vi "ESP301.vi"() -> ()   [LabVIEW 2019]
uses:
  Newport ESP301/Newport ESP301.lvlib
panel:
  in  "DigNum Refnum":refnum<vi>
  out "Numeric":i32
  out "Left Travel Limit (units)":dbl format="%.6g"
  out "Right Travel Limit (units)":dbl format="%.6g"
  in  "Power Status":bool
  out "Units":T1(ring)
  in  "Target position (units)":dbl
  in  "Stop":bool
  out "Position (units)":dbl format="%.6g"
  out "Home High Speed (units/s)":dbl format="%.4g"
  out "Maximum Velocity (units/s)":dbl format="%.4g"
  out "Velocity (units/s)":dbl format="%.4g"
  in  "VISA resource name":refnum<visa-resource-name>
  in  "Axis (1)":i32=1 min=1 max=3
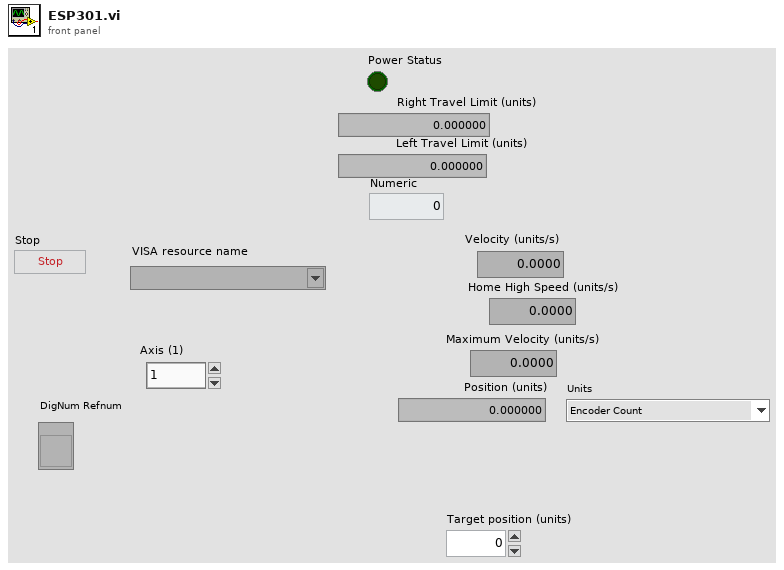
[diagram p1: front panel]
types:
  T1 = enum16{"Encoder Count", "Motor Step", "millimeter", "micrometer", "inch", "milli-inch", "micro-inch", "degree", "gradian", "radian", "milliradian", "microradian"}
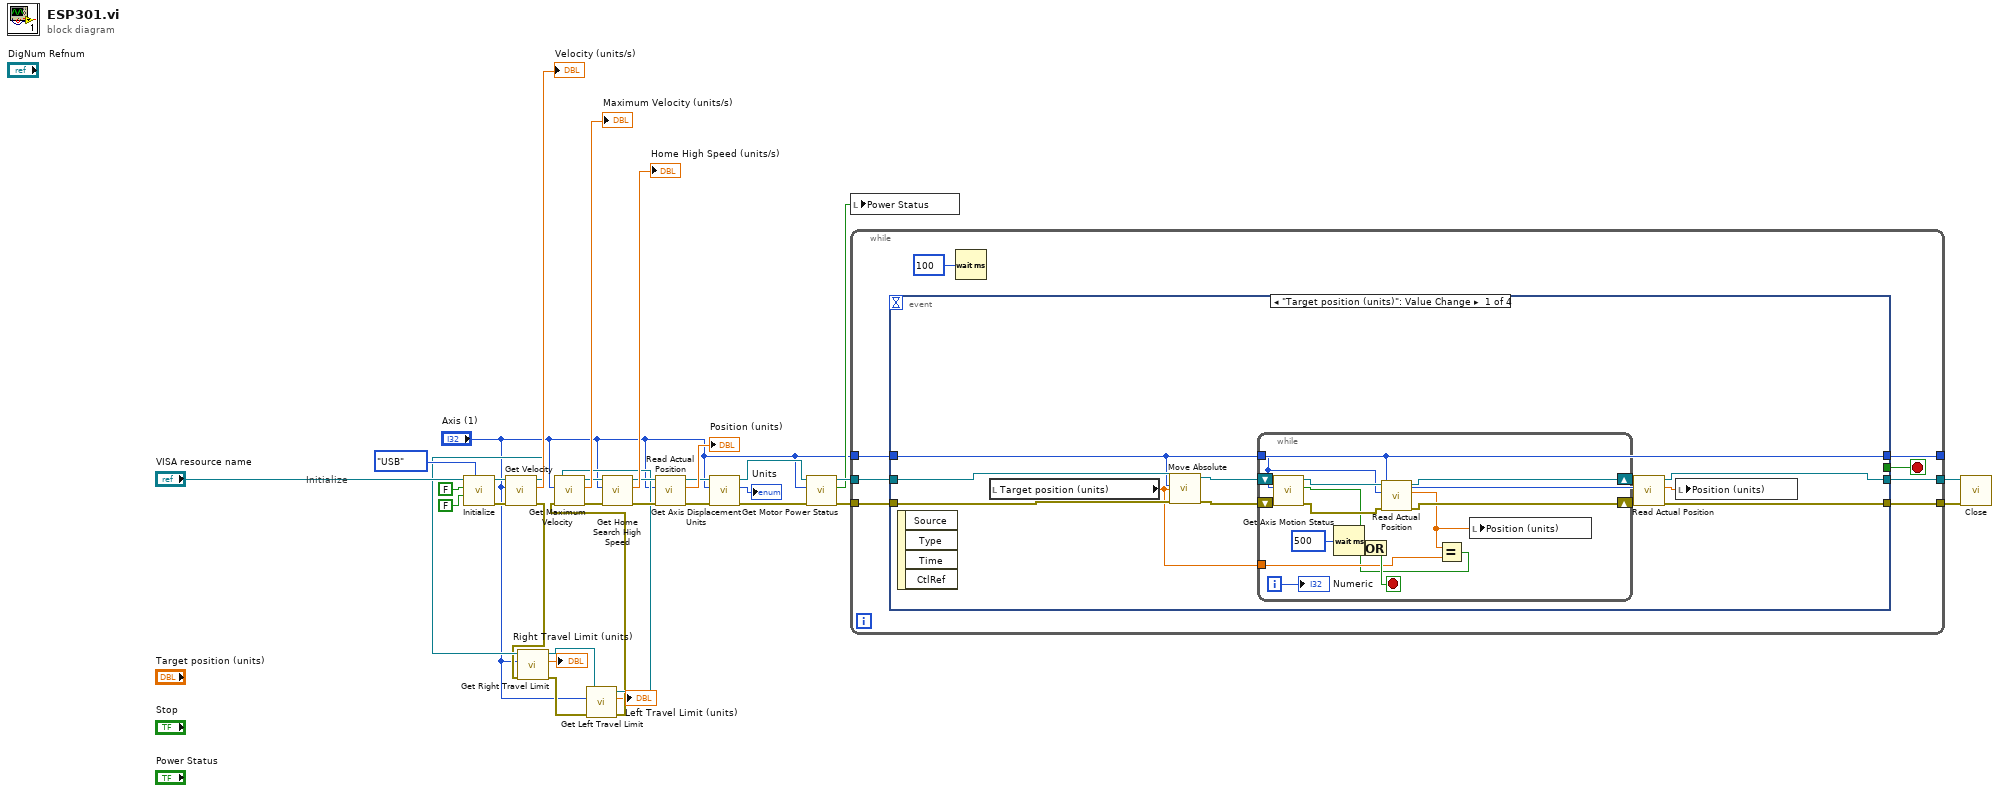
[diagram p0: block diagram]
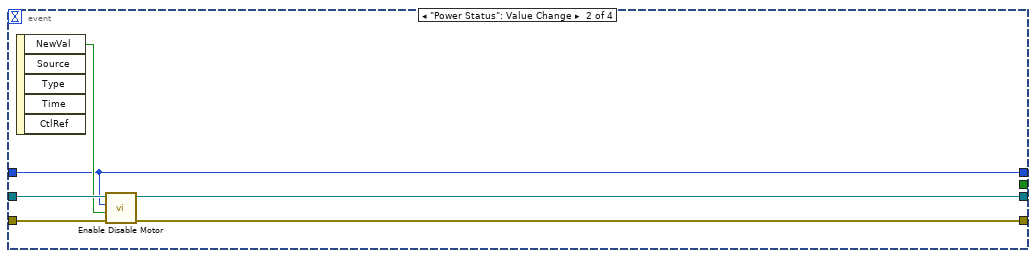
[diagram p2: hidden frame]
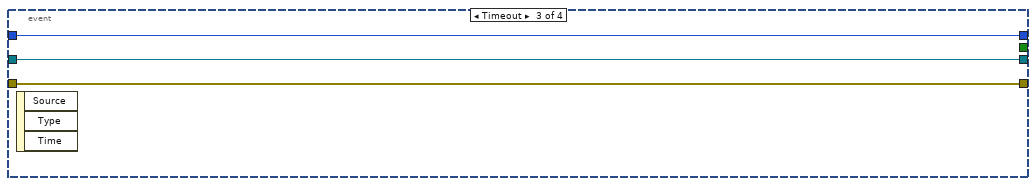
[diagram p3: hidden frame]
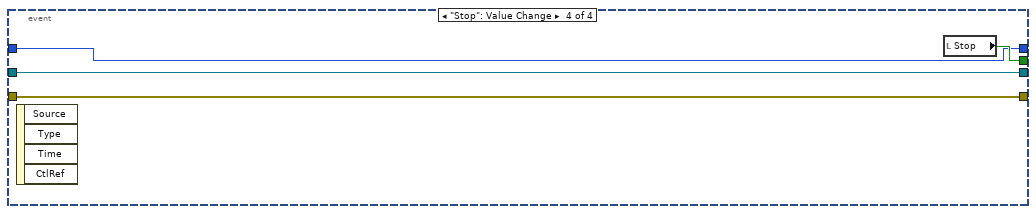
[diagram p4: hidden frame]
diagram:
  # "Initialize"
  n1 = call "Initialize.vi"("VISA resource name"="VISA resource name", "ID Query (True)"=FALSE, "Reset (False)"=FALSE, "Serial Link (RS232)"=enum16{"RS232", "USB"}."USB") -> ("VISA resource name out"=w32:refnum<visa-resource-name>, "error out"=w31:errorcluster)  [unwired: 5 in]
  n2 = call "Get Velocity.vi"("error in (no error)"=w31, "Axis (1)"="Axis (1)", "VISA resource name"=w32) -> ("error out"=w8:errorcluster, "Velocity (units/s)"=→"Velocity (units/s)":dbl, "VISA resource name out"=w9:refnum<visa-resource-name>)  [unwired: 2 in]
  n3 = call "Get Right Travel Limit.vi"("error in (no error)"=w8, "Axis (1)"="Axis (1)", "VISA resource name"=w9) -> ("error out"=w5:errorcluster, "Right Travel Limit (units)"=→"Right Travel Limit (units)":dbl, "VISA resource name out"=w6:refnum<visa-resource-name>)  [unwired: 2 in]
  n4 = call "Get Left Travel Limit.vi"("error in (no error)"=w5, "Axis (1)"="Axis (1)", "VISA resource name"=w6) -> ("error out"=w3:errorcluster, "Left Travel Limit (units)"=→"Left Travel Limit (units)":dbl, "VISA resource name out"=w4:refnum<visa-resource-name>)  [unwired: 2 in]
  n5 = call "Get Maximum Velocity.vi"("error in (no error)"=w3, "Axis (1)"="Axis (1)", "VISA resource name"=w4) -> ("error out"=w28:errorcluster, "Maximum Velocity (units/s)"=→"Maximum Velocity (units/s)":dbl, "VISA resource name out"=w27:refnum<visa-resource-name>)  [unwired: 2 in]
  n6 = call "Get Home Search High Speed.vi"("error in (no error)"=w28, "Axis (1)"="Axis (1)", "VISA resource name"=w27) -> ("error out"=w25:errorcluster, "Home High Speed (units/s)"=→"Home High Speed (units/s)":dbl, "VISA resource name out"=w24:refnum<visa-resource-name>)  [unwired: 2 in]
  n7 = call "Read Actual Position.vi"("error in (no error)"=w25, "Axis (1)"="Axis (1)", "VISA resource name"=w24) -> ("error out"=w22:errorcluster, "Position (units)"=→"Position (units)":dbl, "VISA resource name out"=w21:refnum<visa-resource-name>)  [unwired: 2 in]
  n8 = call "Get Axis Displacement Units.vi"("error in (no error)"=w22, "Axis (1)"="Axis (1)", "VISA resource name"=w21) -> ("error out"=w17:errorcluster, "Units"=→"Units":T1, "VISA resource name out"=w19:refnum<visa-resource-name>)  [unwired: 2 in]
  n9 = call "Get Motor Power Status.vi"("error in (no error)"=w17, "Axis (1)"="Axis (1)", "VISA resource name"=w19) -> ("error out"=w16:errorcluster, "Power Status"=w15:bool, "VISA resource name out"=w18:refnum<visa-resource-name>)  [unwired: 2 in]
  n10 = local write "Power Status"(w15) -> ()
  n11 = while {
    tunnel: w16 -> [w41]
    tunnel: w18 -> [w40]
    tunnel: "Axis (1)" -> [w39]
    tunnel: [w36] -> w10
    tunnel: [w35] -> _
    tunnel: [w34] -> w11
    stop <- w37 stop-if-true
    n12 = event shown="[0] \"Target position (units)\": Value Change" {
      selector: _ -> [_ _ _ _]
      dyn-events: _ -> [_ _ _ _]
      timeout: _ -> [_ _ _ _]
      tunnel: w41 -> [w52 w71 w73 w76]
      tunnel: w40 -> [w51 w72 w75 w78]
      tunnel: w39 -> [w43 w67 w74 w77]
      tunnel: [w46 w68 w75 w78] -> w34
      tunnel: [w45 w69 w73 w76] -> w36
      tunnel: [w43 w67 w74 w77] -> w35
      tunnel: [_ _ _ w79] -> w37
      event "Target position (units)": Value Change {
        n13 = event-data() -> ()  [unwired: 1 in, 4 out]
        n14 = local read "Target position (units)"() -> (w42:dbl)
        n15 = call "Move Absolute.vi"("error in (no error)"=w52, "Position (0 units)"=w42, "Axis (1)"=w43, "VISA resource name"=w51) -> ("error out"=w49:errorcluster, "VISA resource name out"=w50:refnum<visa-resource-name>)  [unwired: 2 in]
        n16 = while {
          tunnel: w43 -> [w60]
          shift-right: [w59] -> w47
          shift-left: w50 -> [w66]
          shift-right: [w58] -> w48
          shift-left: w49 -> [w65]
          tunnel: w42 -> [w55]
          i -> [w64]
          stop <- w57 stop-if-true
          n17 = call "Get Axis Motion Status.vi"("error in (no error)"=w65, "Axis (1)"=w60, "VISA resource name"=w66) -> ("error out"=w61:errorcluster, "Motion Done"=w56:bool, "VISA resource name out"=w62:refnum<visa-resource-name>)  [unwired: 2 in]
          n18 = Wait (ms)(milliseconds to wait=u32 500) -> ()  [unwired: 1 out]
          n19 = call "Read Actual Position.vi"("error in (no error)"=w61, "Axis (1)"=w60, "VISA resource name"=w62) -> ("error out"=w58:errorcluster, "Position (units)"=w53:dbl, "VISA resource name out"=w59:refnum<visa-resource-name>)  [unwired: 2 in]
          n20 = Equal?(x=w53, y=w55) -> (x = y?=w54:bool)
          n21 = Or(x=w56, y=w54) -> (x .or. y?=w57:bool)
          n22 = local write "Position (units)"(w53) -> ()
          "Numeric" <- w64
        }
        n23 = call "Read Actual Position.vi"("error in (no error)"=w48, "Axis (1)"=w43, "VISA resource name"=w47) -> ("error out"=w45:errorcluster, "Position (units)"=w44:dbl, "VISA resource name out"=w46:refnum<visa-resource-name>)  [unwired: 2 in]
        n24 = local write "Position (units)"(w44) -> ()
      }
      event "Power Status": Value Change {
        n25 = event-data() -> ("NewVal"=w70:bool)  [unwired: 1 in, 4 out]
        n26 = call "Enable Disable Motor.vi"("error in (no error)"=w71, "Action (F - OFF)"=w70, "Axis (1)"=w67, "VISA resource name"=w72) -> ("error out"=w69:errorcluster, "VISA resource name out"=w68:refnum<visa-resource-name>)  [unwired: 2 in]
      }
      event Timeout {
        n27 = event-data() -> ()  [unwired: 1 in, 3 out]
      }
      event "Stop": Value Change {
        n28 = event-data() -> ()  [unwired: 1 in, 4 out]
        n29 = local read "Stop"() -> (w79:bool)
      }
    }
    n30 = Wait (ms)(milliseconds to wait=u32 100) -> ()  [unwired: 1 out]
  }
  n31 = call "Close.vi"("error in (no error)"=w10, "VISA resource name"=w11) -> ()  [unwired: 9 in, 1 out]
